vi "Registration Console.vi"(7 "Module Name":string="Module") -> ()   [LabVIEW 2017, in "DebugConsole.lvlib"]
uses:
  DebugConsole.lvlib
  _csmlite/_PassAllowedMessage - Mapping.vi
  _Polymophic/Build Unregister Message.vi
  _csmlite/_csmlite.lvlib
  Communicable State Machine.lvlib
  _ui/csm-ui-support.lvlib
panel:
  in  "Drop All":bool
  in  "Type":enum32{"Rules", "Mapping"}(radio)
  in  "Refresh API":bool
  out "RegistryList":string[][](table)
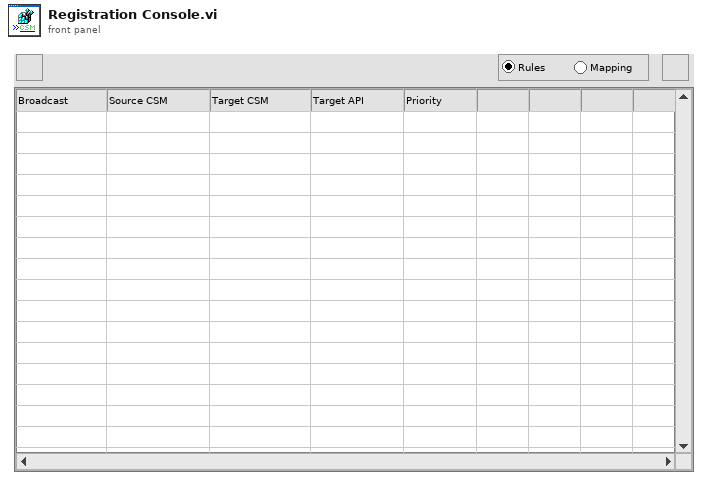
[diagram p1: front panel]
types:
  T1 = enum32{"Invalid", "Standard", "Closed", "Hidden", "Minimized", "Maximized"}
  T2 = enum32{"invalid app kind", "Development System", "Run Time System", "Student Edition", "Embedded LabVIEW", "Evaluation", "Custom"}
  T3 = typedef "LVPoint32TypeDef.ctl" = cluster{"Horizontal":i32, "Vertical":i32}
  T4 = typedef "LVRowAndColumnTypeDef.ctl" = cluster{"Row":i32, "Column":i32}
  T5 = cluster{"Core":cluster{"Current VI Reference":refnum<vi>, "Close Panel on Exit?":bool}, "Your Boolean data":bool, "Your string data":string}
  T6 = cluster{"Current VI Reference":refnum<vi>, "Close Panel on Exit?":bool}
  T7 = typedef "Communicable State Machine.lvlib/CSM - Broadcast Message Type.ctl" = enum16{"<Null>", "Status", "Interrupt"}
  T8 = cluster{"Status":string, "Source CSM":string, "Target CSM":string, "Target API":string, "Register Type":T7}[]
  T9 = cluster{string, "Name":string, "Target CSM":string, "Target State":string, "Register Type":T7}[]
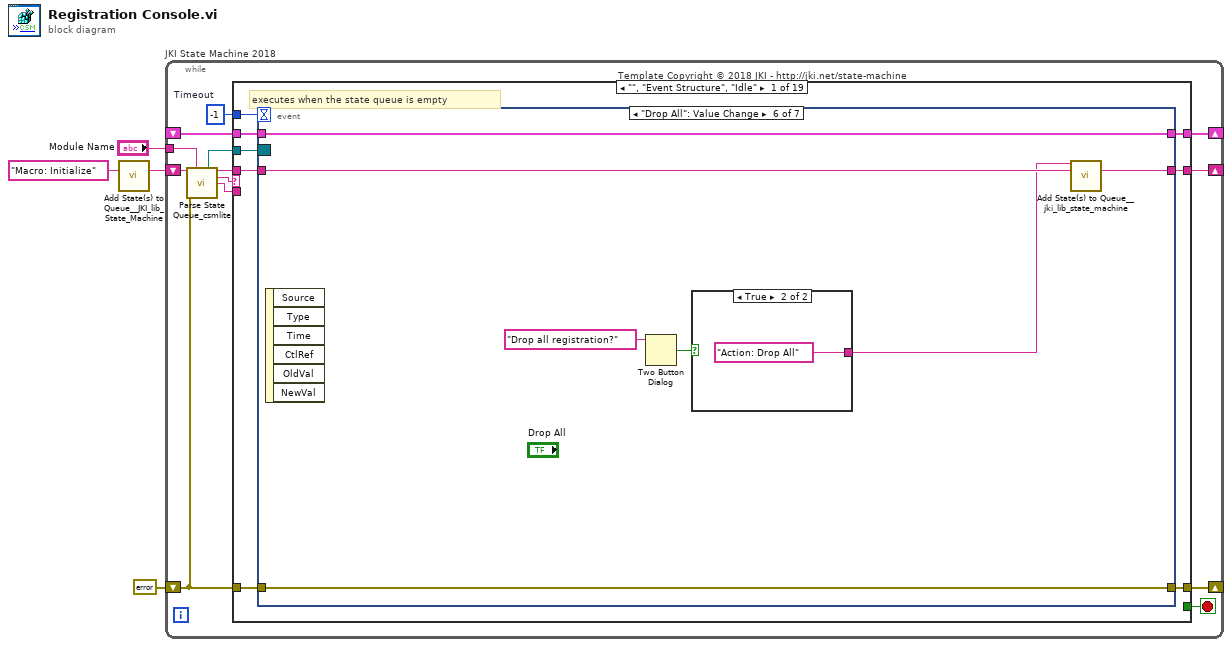
[diagram p0: block diagram]
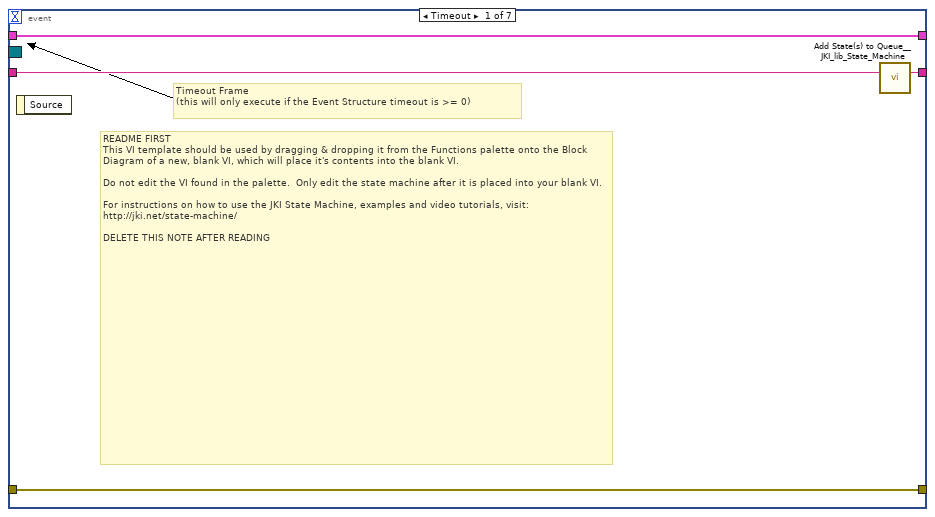
[diagram p2: hidden frame]
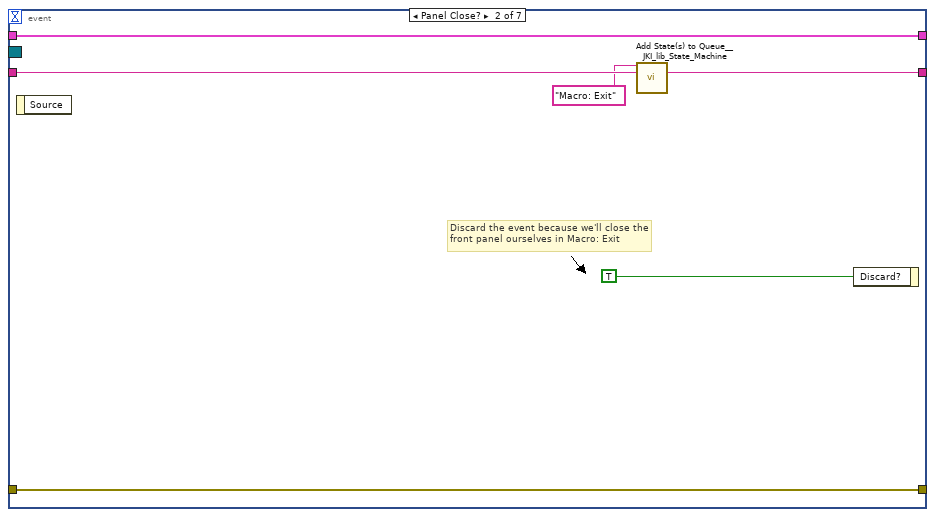
[diagram p3: hidden frame]
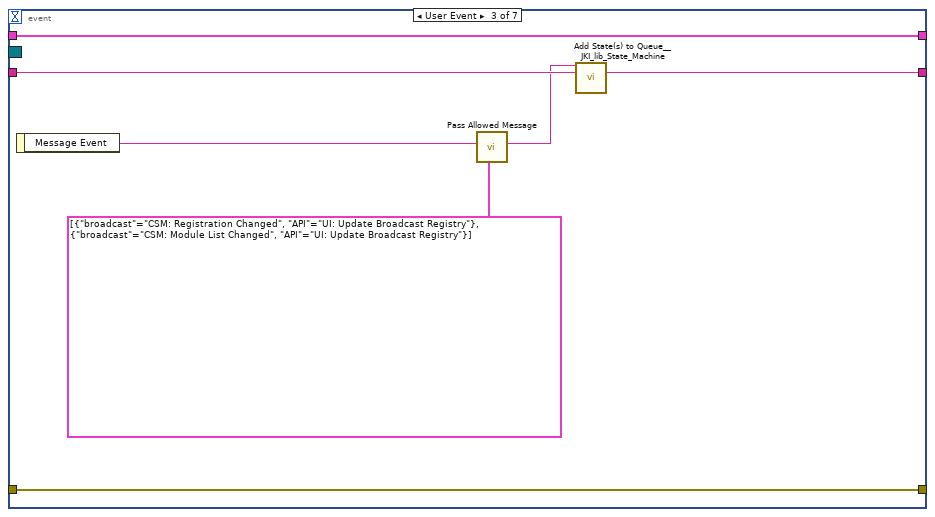
[diagram p4: hidden frame]
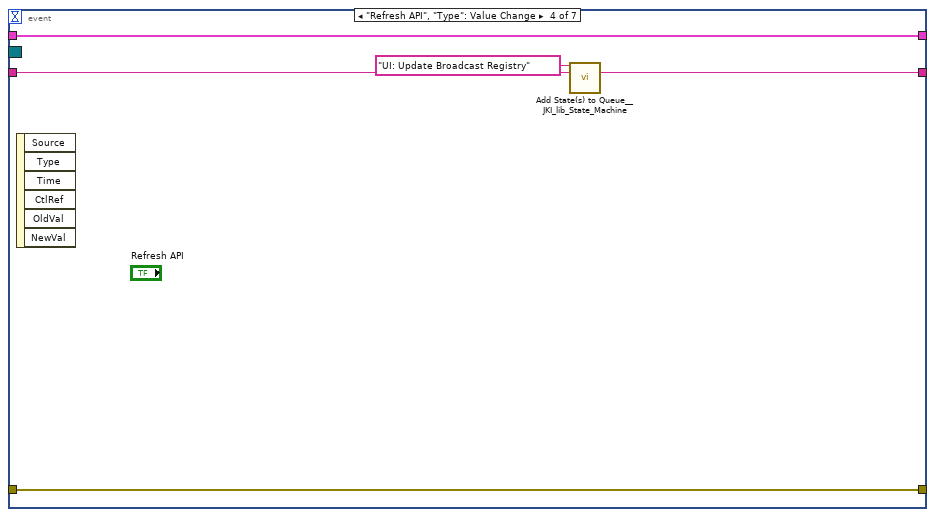
[diagram p5: hidden frame]
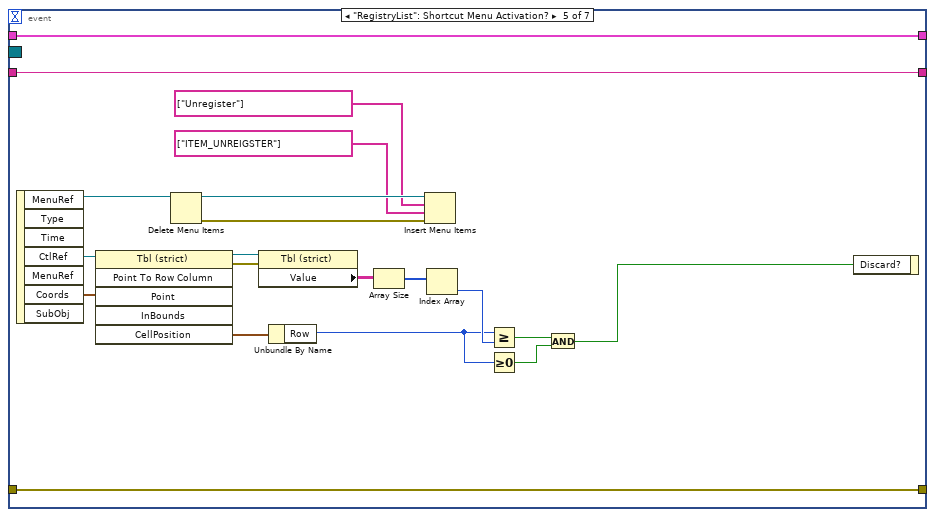
[diagram p6: hidden frame]
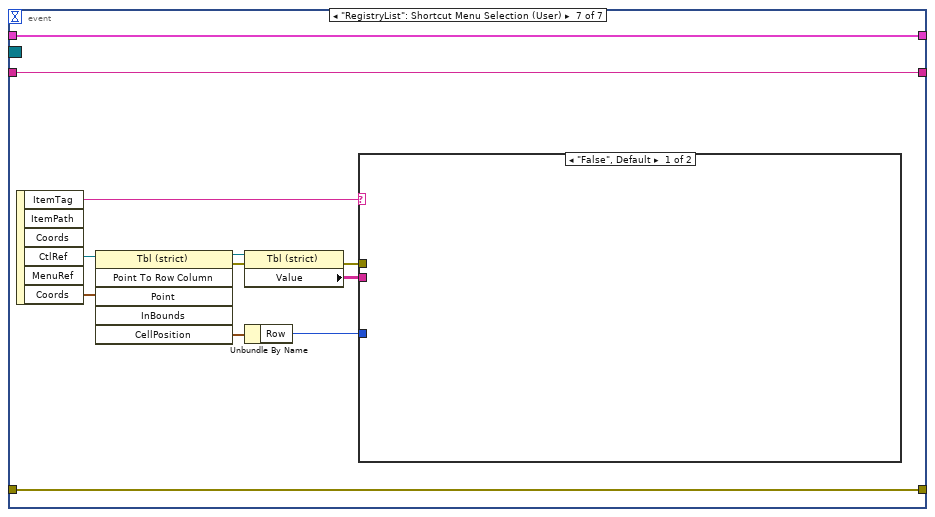
[diagram p8: hidden frame]
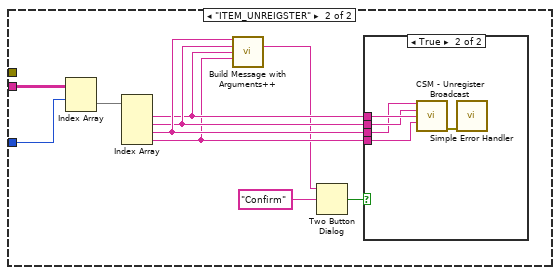
[diagram p9: hidden frame]
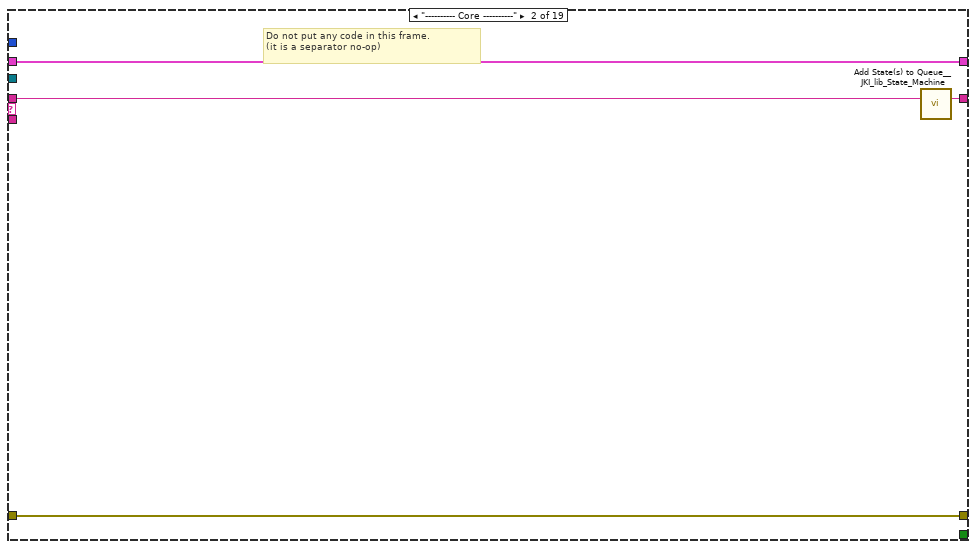
[diagram p11: hidden frame]
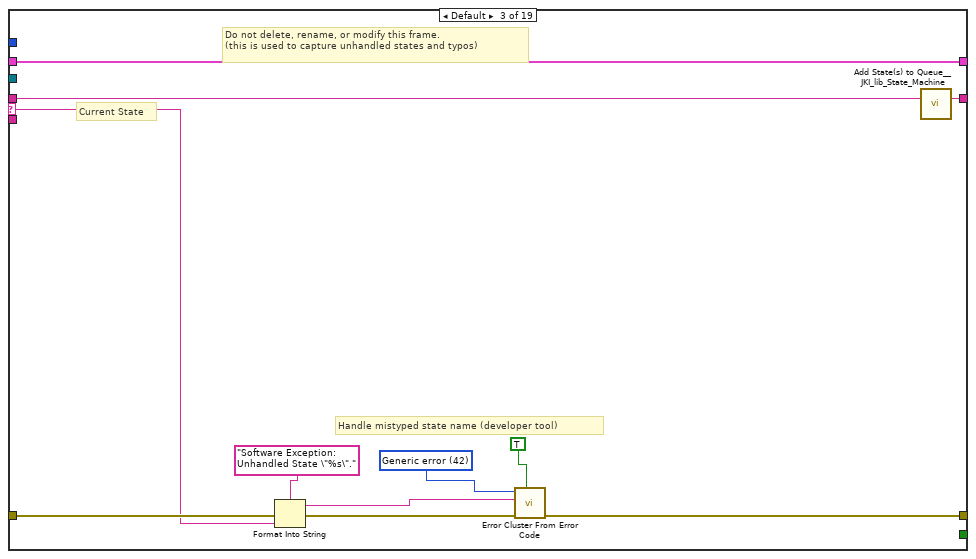
[diagram p12: hidden frame]
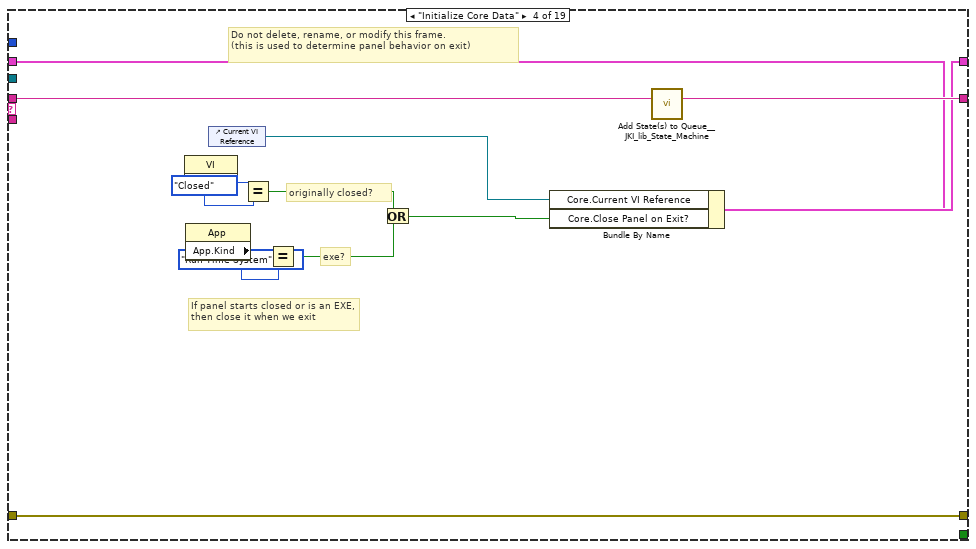
[diagram p13: hidden frame]
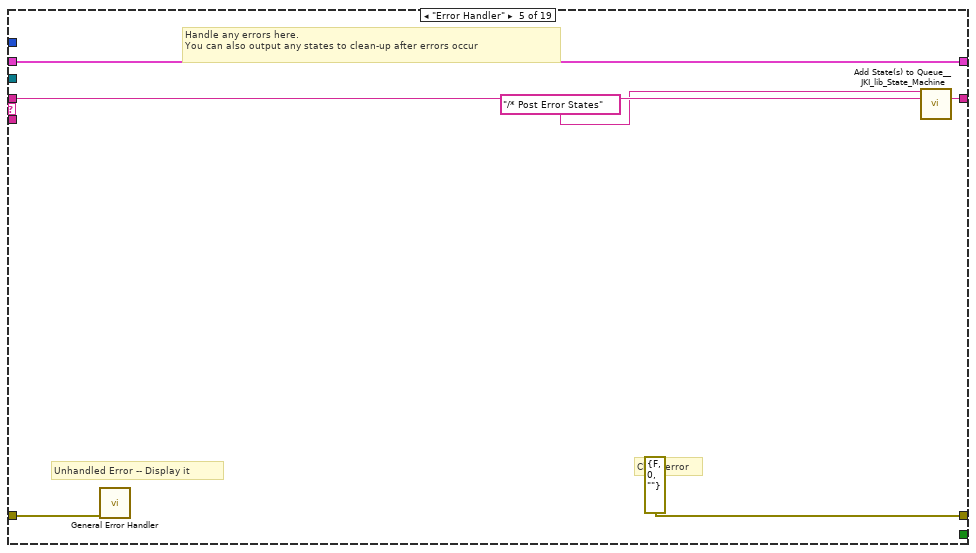
[diagram p14: hidden frame]
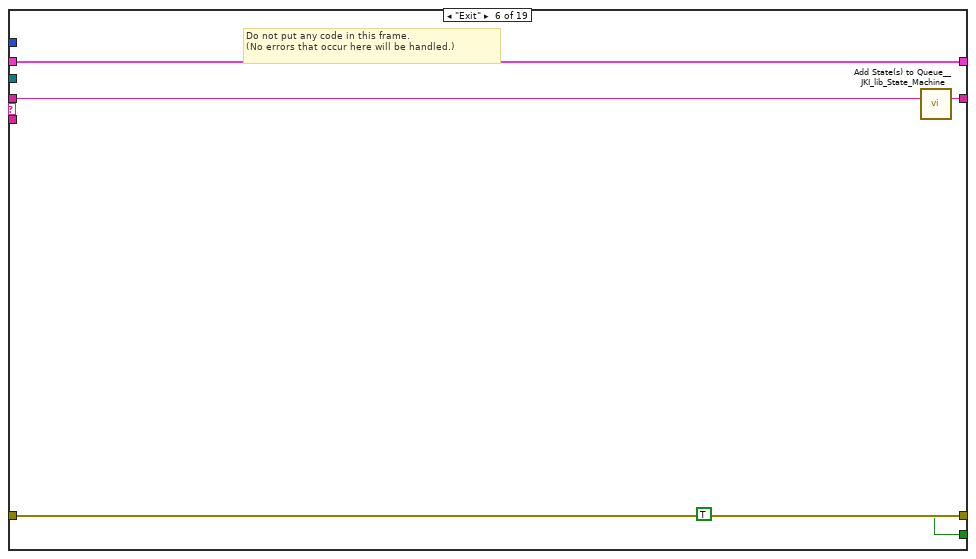
[diagram p15: hidden frame]
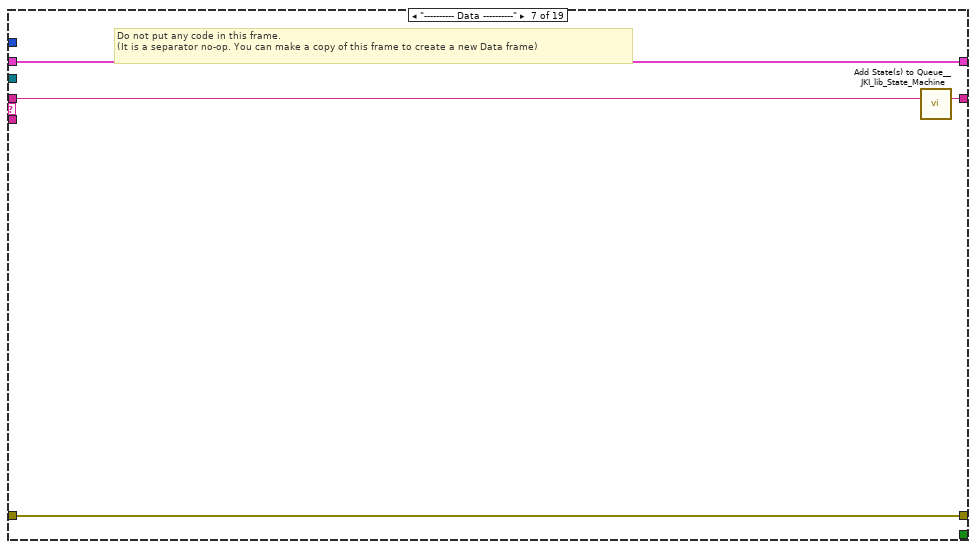
[diagram p16: hidden frame]
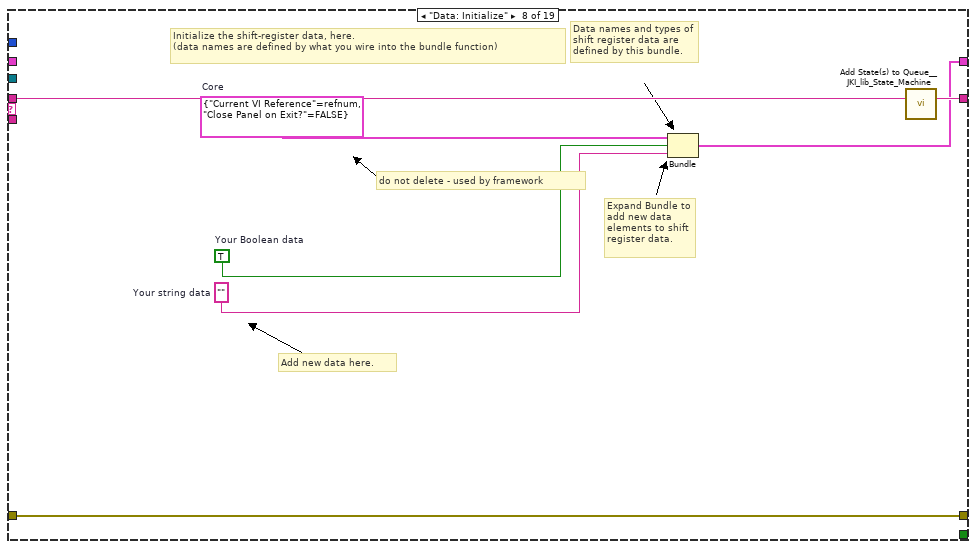
[diagram p17: hidden frame]
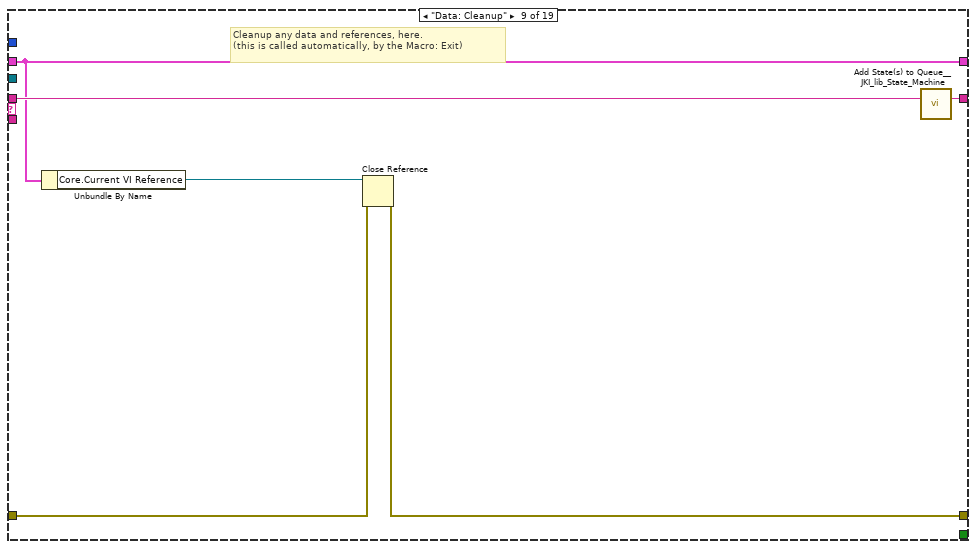
[diagram p18: hidden frame]
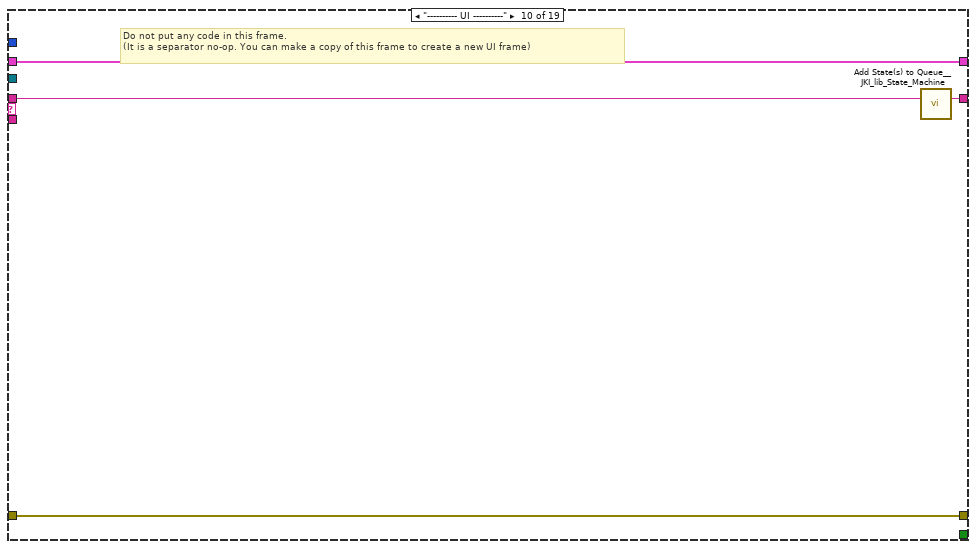
[diagram p19: hidden frame]
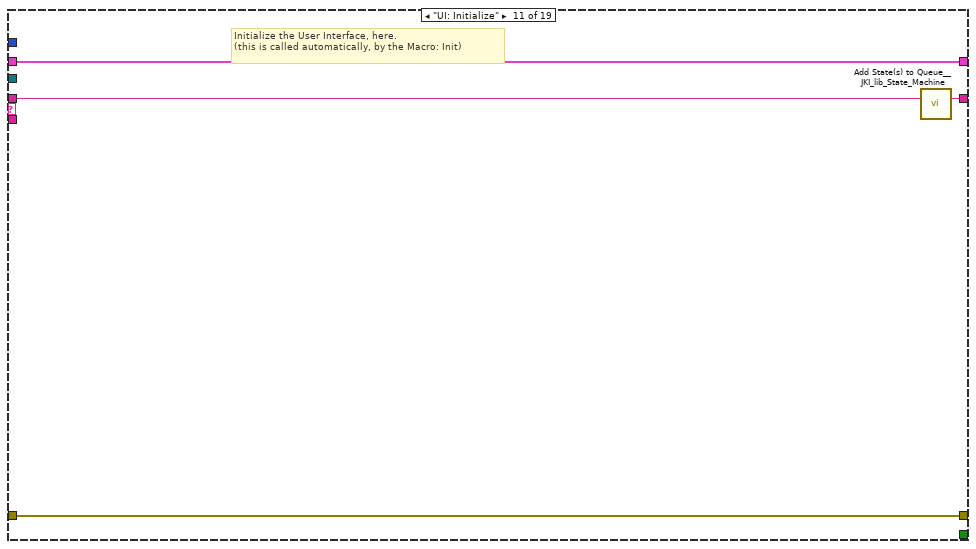
[diagram p20: hidden frame]
diagram:
  n1 = call <vilib>:"Add State(s) to Queue__JKI_lib_State_Machine.vi"("State(s) in (\"\")"="Macro: Initialize") -> ("States Out"=w3:string)  [unwired: 14 in]
  n2 = while "JKI State Machine 2018" {
    shift-right: [w10] -> _
    shift-left: _ -> [w9]
    shift-right: [w13] -> _
    shift-left: errorcluster {"status"=FALSE, "code"=0, "source"=""} ("error out") -> [w7]
    shift-right: [w12] -> _
    shift-left: w3 -> [w14]
    tunnel: "Module Name" -> [w6]
    stop <- w11 stop-if-true
    w8 = -1  # Timeout
    # "Template Copyright © 2018 JKI - http://jki.net/state-machine"
    n3 = call "Parse State Queue_csmlite.vi"("State Queue"=w14, "Current Module(\"\" to generate an ID)"=w6, "Error In (no error)"=w7) -> ("Event Registration Refnum"=w5:refnum<event-registration>, "Remaining States"=w16:string, "Current State"=w17:string, "Arguments"=w15:string)  [unwired: 9 in]
    n4 = case shown="\"\", \"Event Structure\", \"Idle\"" w17 {
      selector: w17 -> [_ _ w107 _ _ _ _ _ _ _ _ _ _ _ _ _ _ _ _]
      tunnel: w16 -> [w25 w106 w111 w130 w136 w141 w145 w152 w158 w162 w166 w172 w183 w259 w273 w278 w288 w292 w294]
      tunnel: w15 -> [_ _ _ _ _ _ _ _ _ _ _ w167 w177 _ _ _ _ _ _]
      tunnel: w9 -> [w23 w103 w109 w123 w133 w139 w142 _ w153 w159 w164 w170 w179 w256 w270 w275 w285 w289 w293]
      tunnel: [w22 w104 w113 w127 errorcluster {"status"=FALSE, "code"=0, "source"=""} ("error out") w138 w143 w149 w154 w160 w163 w168 w180 w257 w271 w276 w286 w290 w295] -> w13
      tunnel: w7 -> [w21 w104 w112 w127 w132 w138 w143 w149 w155 w160 w163 w169 w181 w257 w271 w276 w286 w290 w295]
      tunnel: [w24 w105 w110 w129 w135 w140 w144 w151 w157 w161 w165 w171 w182 w258 w272 w277 w287 w291 w294] -> w12
      tunnel: [_ _ _ _ _ TRUE _ _ _ _ _ _ _ _ _ _ _ _ _] -> w11
      tunnel: [w20 w103 w109 w128 w133 w139 w142 w150 w153 w159 w164 w170 w179 w256 w270 w275 w285 w289 w293] -> w10
      tunnel: w8 -> [w19 _ _ _ _ _ _ _ _ _ _ _ _ _ _ _ _ _ _]
      tunnel: w5 -> [w18 _ _ _ _ _ _ _ _ _ _ _ _ _ _ _ _ _ _]
      frame "", "Event Structure", "Idle" {
        # "executes when the state queue is empty"
        n5 = event shown="[5] \"Drop All\": Value Change" {
          selector: w18 -> [_ _ _ _ _ _ _]
          dyn-events: _ -> [_ _ _ _ _ _ _]
          timeout: w19 -> [_ _ _ _ _ _ _]
          tunnel: w25 -> [w29 w35 w40 w44 w67 w71 w87]
          tunnel: [w28 w34 w38 w45 w67 w72 w87] -> w24
          tunnel: w23 -> [w26 w32 w41 w46 w65 w73 w85]
          tunnel: [w27 w33 w42 w47 w66 w74 w86] -> w22
          tunnel: w21 -> [w27 w33 w42 w47 w66 w74 w86]
          tunnel: [w26 w32 w41 w46 w65 w73 w85] -> w20
          event Timeout {
            # "README FIRST\nThis VI template should be used by dragging & dropping it from the Functions palette onto the Block Diagram of a new, blank VI, which will place it's contents into the blank VI.\n\nDo not edit the VI found in the palette.  Only edit the state machine after it is placed into your blank VI.\n\nFor instructions on how to use the JKI State Machine, examples and video tutorials, visit:\nhttp://jki.net/state-machine/\n\nDELETE THIS NOTE AFTER READING"
            # "Timeout Frame\n(this will only execute if the Event Structure timeout is >= 0)"
            n6 = event-data() -> ()  [unwired: 1 in, 1 out]
            n7 = call <vilib>:"Add State(s) to Queue__JKI_lib_State_Machine.vi"("State(s) in (\"\")"=w29) -> ("States Out"=w28:string)  [unwired: 14 in]
          }
          event Panel Close? {
            # "Discard the event because we'll close the front panel ourselves in Macro: Exit"
            n8 = event-data() -> ()  [unwired: 1 in, 1 out]
            n9 = call <vilib>:"Add State(s) to Queue__JKI_lib_State_Machine.vi"("State(s) in Front (\"\")"="Macro: Exit", "State(s) in (\"\")"=w35) -> ("States Out"=w34:string)  [unwired: 13 in]
            n10 = event-data("Discard?"=TRUE) -> ()  [unwired: 1 in, 1 out]
          }
          event User Event {
            n11 = event-data() -> ("Message Event"=w39:string)  [unwired: 1 in]
            n12 = call-poly "Pass Allowed Message.vi"("Mapping"=cluster{"broadcast":string, "API":string}[] [{"broadcast"="CSM: Registration Changed", "API"="UI: Update Broadcast Registry"}, {"broadcast"="CSM: Module List Changed", "API"="UI: Update Broadcast Registry"}], "JKISM External Event"=w39) -> ("States"=w37:string)  [unwired: 7 in]
            n13 = call <vilib>:"Add State(s) to Queue__JKI_lib_State_Machine.vi"("State(s) in Front (\"\")"=w37, "State(s) in (\"\")"=w40) -> ("States Out"=w38:string)  [unwired: 13 in]
          }
          event "Refresh API", "Type": Value Change {
            n14 = event-data() -> ()  [unwired: 1 in, 6 out]
            n15 = call <vilib>:"Add State(s) to Queue__JKI_lib_State_Machine.vi"("State(s) in Front (\"\")"="UI: Update Broadcast Registry" ("State(s) in Front (\"\")"), "State(s) in (\"\")"=w44) -> ("States Out"=w45:string)  [unwired: 13 in]
          }
          event "RegistryList": Shortcut Menu Activation? {
            n16 = event-data() -> ("MenuRef"=w58:refnum<k9>, "CtlRef"=w64:refnum<vi>, "Coords"=w63:T3)  [unwired: 1 in, 4 out]
            n17 = invoke class="Tbl (strict)" method="Point To Row Column"(reference=w64, "Point"=w63) -> (reference out=w62:refnum<vi>, error out=w61:errorcluster, "CellPosition"=w60:T4)  [unwired: 4 in, 3 out]
            n18 = Delete Menu Items(9:w58) -> (0:w57:errorcluster, 3:w56:refnum<k9>)  [unwired: 3 in]
            n19 = property class="Tbl (strict)"(reference=w62, error in=w61) -> ("Value"=w59:string[][])  [unwired: 2 out]
            n20 = Unbundle By Name(w60) -> ("Row"=w49:i32)
            n21 = Array Size(array=w59) -> (size(s)=w53:i32[])
            n22 = Insert Menu Items(6:w57, 7:string[] ["ITEM_UNREIGSTER"] ("item names"), 8:string[] ["Unregister"] ("item names"), 9:w56) -> ()  [unwired: 2 in, 3 out]
            n23 = Index Array(array=w53) -> (element=w52:i32)  [unwired: 1 in]
            n24 = Greater Or Equal?(x=w49, y=w52) -> (x >= y?=w51:bool)
            n25 = Greater Or Equal To 0?(x=w49) -> (x >= 0?=w48:bool)
            n26 = And(x=w51, y=w48) -> (x .and. y?=w50:bool)
            n27 = event-data("Discard?"=w50) -> ()  [unwired: 1 in, 1 out]
          }
          event "Drop All": Value Change {
            n28 = event-data() -> ()  [unwired: 1 in, 6 out]
            n29 = Two Button Dialog(message="Drop all registration?") -> (T button?=w69:bool)  [unwired: 2 in]
            n30 = case shown="True" w69 {
              tunnel: [_ "Action: Drop All" ("State(s) in Front (\"\")")] -> w70
              frame False {
              }
              frame True {
              }
            }
            n31 = call <vilib>:"Add State(s) to Queue__jki_lib_state_machine.vi"("State(s) in Front (\"\")"=w70, "State(s) in (\"\")"=w71) -> ("States Out"=w72:string)  [unwired: 13 in]
          }
          event "RegistryList": Shortcut Menu Selection (User) {
            n32 = event-data() -> ("ItemTag"=w79:string, "CtlRef"=w84:refnum<vi>, "Coords"=w83:T3)  [unwired: 1 in, 3 out]
            n33 = invoke class="Tbl (strict)" method="Point To Row Column"(reference=w84, "Point"=w83) -> (reference out=w82:refnum<vi>, error out=w81:errorcluster, "CellPosition"=w80:T4)  [unwired: 4 in, 3 out]
            n34 = property class="Tbl (strict)"(reference=w82, error in=w81) -> (error out=w78:errorcluster, "Value"=w77:string[][])  [unwired: 1 out]
            n35 = Unbundle By Name(w80) -> ("Row"=w76:i32)
            n36 = case shown="\"False\", Default" w79 {
              tunnel: w78 -> [_ _]
              tunnel: w77 -> [_ w97]
              tunnel: w76 -> [_ w96]
              frame "False", Default {
              }
              frame "ITEM_UNREIGSTER" {
                n37 = Index Array(array=w97, index (row)=w96) -> (element=w95:string[])  [unwired: 1 in]
                n38 = Index Array(array=w95) -> (element #1=w91:string, element #2=w92:string, element #3=w93:string, element #4=w90:string)  [unwired: 4 in]
                n39 = call-poly "Build Message with Arguments++.vi"("Target CSM"=w93, "Source CSM (* as Default)"=w92, "Status"=w91, "API (* as Default)"=w90) -> ("CSM Message String"=w88:string)  [unwired: 11 in]
                n40 = Two Button Dialog(message=w88, 2:"Confirm" ("message")) -> (T button?=w94:bool)  [unwired: 1 in]
                n41 = case shown="True" w94 {
                  tunnel: w91 -> [_ w101]
                  tunnel: w92 -> [_ w100]
                  tunnel: w93 -> [_ w99]
                  tunnel: w90 -> [_ w98]
                  frame False {
                  }
                  frame True {
                    n42 = call "CSM - Unregister Broadcast.vi"("CSM Name(Empty for Broadcast Event)"=w99, "Source CSM Name (* as Default)"=w100, "Trigger"=w101, "API (\"*\" as Default)"=w98) -> ("error out"=w102:errorcluster)  [unwired: 10 in, 1 out]
                    n43 = call <vilib>:"Simple Error Handler.vi"("error in (no error)"=w102) -> ()  [unwired: 4 in, 5 out]
                  }
                }
              }
            }
          }
        }
      }
      frame "---------- Core ----------" {
        # "Do not put any code in this frame.\n(it is a separator no-op)"
        n44 = call <vilib>:"Add State(s) to Queue__JKI_lib_State_Machine.vi"("State(s) in (\"\")"=w106) -> ("States Out"=w105:string)  [unwired: 14 in]
      }
      frame Default {
        w116 = 42 items=["No error", "Argument error", "Memory is full", "Out of zone", "End of file", "File already open", "Generic file I/O error", "File not found", "File permission error", "Disk is full", "Duplicate path", "Too many files open", "System feature not enabled", "Resource file not found", "Cannot add resource", "Resource not found", "Image not found", "Image memory error", "Pen does not exist", "Config type invalid", "Config token not found", "Config parse error", "Config memory error", "Bad external code format", "Bad external code offset", "External code not present", "Null window", "Destroy window error", "Null menu", "Print aborted", "Bad print record", "Print driver error", "Windows error during printing", "Memory error during printing", "Print dialog error", "Generic print error", "Invalid device refnum", "Device not found", "Device parameter error", "Device unit error", "Cannot open device", "Device call aborted", "Generic error", "Cancelled by user", "Object ID too low", "Object ID too high", "Object not in heap", "Unknown heap", "Unknown object (invalid DefProc)", "Unknown object (DefProc not in table)", "Message out of range", "Invalid (null) method", "Unknown message", "Manager call not supported", "Bad address", "Network operation in progress", "Network operation timed out", "Connection is busy", "Network attribute not supported", "Network error", "Address in use", "System out of memory", "Connection aborted", "Connection refused", "Not connected", "Already connected", "Connection closed", "Initialization error (interapplication manager)", "Bad occurrence", "Wait on unbound occurrence handler", "Occurrence queue overflow", "Datalog type conflict", "Unused", "Unrecognized type (interapplication manager)", "Memory corrupt", "Failed to make temporary DLL", "Old CIN version", "Drag socket not found", "Failed to load drop-object", "Failed to register OLE object", "Failed to release OLE object", "Format specifier type mismatch", "Unknown format specifier", "Too few format specifiers", "Too many format specifiers", "Scan failed", "Newer CIN version", "Error converting to variant", "Runtime menu error", "Password tampered", "Variant attribute not found", "Incompatible variant data type", "Event data is not available", "Event Store is not present", "Occurrence is not found", "Event Queue is not created", "Event info is not available", "Refnum passed is NULL", "Error retrieving Class GUID", "Error retrieving CoClass GUID", "Error retrieving TypeLib GUID.", "Bad built application magic bytes.", "Specific driver is different from the specific driver associated with the Logical Name.", "There is no session opened to the class driver.", "Max Error", "MAX - Error with config objects", "MAX - Error loading configuration", "MAX - Group not supported"]
        # "Current State"
        # "Do not delete, rename, or modify this frame.\n(this is used to capture unhandled states and typos)"
        # "Handle mistyped state name (developer tool)"
        n45 = Format Into String(format string="Software Exception: Unhandled State \"%s\"." ("message"), error in=w112, w107) -> (resulting string=w115:string, error out=w114:errorcluster)  [unwired: 1 in]
        n46 = call <vilib>:"Error Cluster From Error Code.vi"("show call chain? (False)"=TRUE, "error in (no error)"=w114, "error message (\"\")"=w115, "error code (0)"=w116) -> ("error out"=w113:errorcluster)  [unwired: 5 in]
        n47 = call <vilib>:"Add State(s) to Queue__JKI_lib_State_Machine.vi"("State(s) in (\"\")"=w111) -> ("States Out"=w110:string)  [unwired: 14 in]
      }
      frame "Initialize Core Data" {
        # "Do not delete, rename, or modify this frame.\n(this is used to determine panel behavior on exit)"
        # "originally closed?"
        # "exe?"
        # "If panel starts closed or is an EXE, then close it when we exit"
        n48 = property class="VI"() -> ("FP.State"=w120:T1)  [unwired: 2 in, 2 out]
        n49 = property class="App"() -> ("App.Kind"=w126:T2)  [unwired: 2 in, 2 out]
        n50 = control-ref of="Current VI Reference"() -> (w121:refnum<vi>)
        n51 = Equal?(x=w120, y=T1."Closed" ("Front Panel Window:State")) -> (x = y?=w118:bool)
        n52 = Equal?(x=w126, y=T2."Run Time System" ("Application:Kind")) -> (x = y?=w124:bool)
        n53 = Or(x=w118, y=w124) -> (x .or. y?=w122:bool)
        n54 = Bundle By Name(cluster=w123, "Core.Current VI Reference"=w121, "Core.Close Panel on Exit?"=w122) -> (w128:T5)
        n55 = call <vilib>:"Add State(s) to Queue__JKI_lib_State_Machine.vi"("State(s) in (\"\")"=w130) -> ("States Out"=w129:string)  [unwired: 14 in]
      }
      frame "Error Handler" {
        # "Unhandled Error -- Display it"
        # "Handle any errors here.\nYou can also output any states to clean-up after errors occur"
        # "Clear error"
        n56 = call <vilib>:"General Error Handler.vi"("error in (no error)"=w132) -> ()  [unwired: 10 in, 5 out]
        n57 = call <vilib>:"Add State(s) to Queue__JKI_lib_State_Machine.vi"("State(s) in Front (\"\")"="/* Post Error States", "State(s) in (\"\")"=w136) -> ("States Out"=w135:string)  [unwired: 13 in]
      }
      frame "Exit" {
        # "Do not put any code in this frame.\n(No errors that occur here will be handled.)"
        n58 = call <vilib>:"Add State(s) to Queue__JKI_lib_State_Machine.vi"("State(s) in (\"\")"=w141) -> ("States Out"=w140:string)  [unwired: 14 in]
      }
      frame "---------- Data ----------" {
        # "Do not put any code in this frame.\n(It is a separator no-op. You can make a copy of this frame to create a new Data frame)"
        n59 = call <vilib>:"Add State(s) to Queue__JKI_lib_State_Machine.vi"("State(s) in (\"\")"=w145) -> ("States Out"=w144:string)  [unwired: 14 in]
      }
      frame "Data: Initialize" {
        w146 = T6 {"Current VI Reference"=refnum, "Close Panel on Exit?"=FALSE}  # Core
        w148 = TRUE  # Your Boolean data
        w147 = ""  # Your string data
        # "do not delete - used by framework"
        # "Expand Bundle to add new data elements to shift register data."
        # "Add new data here."
        # "Data names and types of shift register data are defined by this bundle."
        # "Initialize the shift-register data, here.\n(data names are defined by what you wire into the bundle function)"
        n60 = Bundle("Core"=w146, "Your Boolean data"=w148, "Your string data"=w147) -> (w150:T5)  [unwired: 1 in]
        n61 = call <vilib>:"Add State(s) to Queue__JKI_lib_State_Machine.vi"("State(s) in (\"\")"=w152) -> ("States Out"=w151:string)  [unwired: 14 in]
      }
      frame "Data: Cleanup" {
        # "Cleanup any data and references, here.\n(this is called automatically, by the Macro: Exit)"
        n62 = Unbundle By Name(w153) -> ("Core.Current VI Reference"=w156:refnum<vi>)
        n63 = Close Reference(reference=w156, error in (no error)=w155) -> (error out=w154:errorcluster)
        n64 = call <vilib>:"Add State(s) to Queue__JKI_lib_State_Machine.vi"("State(s) in (\"\")"=w158) -> ("States Out"=w157:string)  [unwired: 14 in]
      }
      frame "---------- UI ----------" {
        # "Do not put any code in this frame.\n(It is a separator no-op. You can make a copy of this frame to create a new UI frame)"
        n65 = call <vilib>:"Add State(s) to Queue__JKI_lib_State_Machine.vi"("State(s) in (\"\")"=w162) -> ("States Out"=w161:string)  [unwired: 14 in]
      }
      frame "UI: Initialize" {
        # "Initialize the User Interface, here.\n(this is called automatically, by the Macro: Init)"
        n66 = call <vilib>:"Add State(s) to Queue__JKI_lib_State_Machine.vi"("State(s) in (\"\")"=w166) -> ("States Out"=w165:string)  [unwired: 14 in]
      }
      frame "UI: Cursor Set" {
        # "Argument"
        # "Set and Unset Cursor Busy.\n(Usage: \"UI: Cursor Set >> Busy|Idle\")"
        n67 = case shown="\"Idle\", Default" w167 {
          tunnel: w169 -> [w174 w176]
          tunnel: [w173 w175] -> w168
          frame "Idle", Default {
            n68 = call <vilib>:"Unset Busy.vi"("error in (no error)"=w174) -> ("error out"=w173:errorcluster)  [unwired: 10 in]
          }
          frame "Busy" {
            n69 = call <vilib>:"Set Busy.vi"("error in (no error)"=w176) -> ("error out"=w175:errorcluster)  [unwired: 9 in, 1 out]
          }
        }
        n70 = call <vilib>:"Add State(s) to Queue__JKI_lib_State_Machine.vi"("State(s) in (\"\")"=w172) -> ("States Out"=w171:string)  [unwired: 14 in]
      }
      frame "UI: Front Panel State" {
        # "Argument"
        # "Set Front Panel Open or Closed\n(Usage: \"UI: Front Panel State >> Open|Close\")"
        n71 = Unbundle By Name(w179) -> ("Core.Current VI Reference"=w178:refnum<vi>)
        n72 = case shown="\"Minimize\", \"Minimized\"" w177 {
          tunnel: w181 -> [w189 w204 w215 w228 w241]
          tunnel: [w191 w205 w217 w230 w243] -> w180
          tunnel: w178 -> [w190 w202 w216 w229 w242]
          frame "Open", "Standard", Default {
            w184 = T1."Standard" ("State")
            n73 = property class="VI"(reference=w190, error in=w189) -> (reference out=w187:refnum<vi>, error out=w188:errorcluster, "FP.State"=w186:T1)
            n74 = Not Equal?(x=w186, y=w184) -> (x != y?=w185:bool)
            n75 = case shown="True" w185 {
              tunnel: [w195 w197] -> w191
              tunnel: w188 -> [w194 w197]
              tunnel: w187 -> [w193 _]
              tunnel: w184 -> [w192 _]
              frame True {
                n76 = invoke class="VI" method="FP.Open"(reference=w193, error in=w194, "Activate"=TRUE, "State"=w192) -> (error out=w195:errorcluster)  [unwired: 1 in, 4 out]
              }
              frame False {
              }
            }
          }
          frame "Close", "Closed" {
            n77 = property class="VI"(reference=w202, error in=w204) -> (reference out=w201:refnum<vi>, error out=w203:errorcluster, "FP.State"=w199:T1)
            n78 = Not Equal?(x=w199, y=T1."Closed" ("Front Panel Window:State")) -> (x != y?=w198:bool)
            n79 = case shown="True" w198 {
              tunnel: [w206 w209] -> w205
              tunnel: w203 -> [w206 w208]
              tunnel: w201 -> [_ w207]
              frame False {
              }
              frame True {
                n80 = invoke class="VI" method="FP.Close"(reference=w207, error in=w208) -> (error out=w209:errorcluster)  [unwired: 1 in, 2 out]
              }
            }
          }
          frame "Hidden", "Hide" {
            w210 = T1."Hidden" ("State")
            n81 = property class="VI"(reference=w216, error in=w215) -> (reference out=w213:refnum<vi>, error out=w214:errorcluster, "FP.State"=w212:T1)
            n82 = Not Equal?(x=w212, y=w210) -> (x != y?=w211:bool)
            n83 = case shown="True" w211 {
              tunnel: [w221 w222] -> w217
              tunnel: w214 -> [w220 w222]
              tunnel: w213 -> [w219 _]
              tunnel: w210 -> [w218 _]
              frame True {
                n84 = invoke class="VI" method="FP.Open"(reference=w219, error in=w220, "State"=w218) -> (error out=w221:errorcluster)  [unwired: 2 in, 4 out]
              }
              frame False {
              }
            }
          }
          frame "Minimize", "Minimized" {
            w223 = T1."Minimized" ("State")
            n85 = property class="VI"(reference=w229, error in=w228) -> (reference out=w226:refnum<vi>, error out=w227:errorcluster, "FP.State"=w225:T1)
            n86 = Not Equal?(x=w225, y=w223) -> (x != y?=w224:bool)
            n87 = case shown="True" w224 {
              tunnel: [w234 w235] -> w230
              tunnel: w227 -> [w233 w235]
              tunnel: w226 -> [w232 _]
              tunnel: w223 -> [w231 _]
              frame True {
                n88 = invoke class="VI" method="FP.Open"(reference=w232, error in=w233, "State"=w231) -> (error out=w234:errorcluster)  [unwired: 2 in, 4 out]
              }
              frame False {
              }
            }
          }
          frame "Maximize", "Maximized" {
            w236 = T1."Maximized" ("State")
            n89 = property class="VI"(reference=w242, error in=w241) -> (reference out=w239:refnum<vi>, error out=w240:errorcluster, "FP.State"=w238:T1)
            n90 = Not Equal?(x=w238, y=w236) -> (x != y?=w237:bool)
            n91 = case shown="True" w237 {
              tunnel: [w247 w248] -> w243
              tunnel: w240 -> [w246 w248]
              tunnel: w239 -> [w245 _]
              tunnel: w236 -> [w244 _]
              frame True {
                n92 = invoke class="VI" method="FP.Open"(reference=w245, error in=w246, "State"=w244) -> (error out=w247:errorcluster)  [unwired: 2 in, 4 out]
              }
              frame False {
              }
            }
          }
        }
        n93 = call <vilib>:"Add State(s) to Queue__JKI_lib_State_Machine.vi"("State(s) in (\"\")"=w183) -> ("States Out"=w182:string)  [unwired: 14 in]
      }
      frame "UI: Update Broadcast Registry" {
        n94 = case shown="\"Rules\", Default" "Type" {
          tunnel: [w260 w261] -> w255
          frame "Rules", Default {
            n95 = call "CSM - List Rules in Broadcast Registry.vi"() -> ("Rule Entries with Register Type"=w260:T8)  [unwired: 9 in, 2 out]
          }
          frame "Mapping" {
            n96 = call "CSM - List Mapping Relationships in Broadcast Registry.vi"() -> ("Mapping Relationships"=w261:T9)  [unwired: 10 in, 1 out]
          }
        }
        n97 = for {
          tunnel: w255 -> [w269] mode=indexing
          tunnel: [w262] -> w254 mode=indexing
          n98 = Unbundle(w269) -> ("Status"=w268:string, "Name"=w267:string, "Target CSM"=w266:string, "Target State"=w265:string, "Register Type"=w264:T7)
          n99 = Format Into String(w264) -> (resulting string=w263:string)  [unwired: 3 in, 1 out]
          n100 = Build Array(w268, w267, w266, w265, w263) -> (w262:string[])
        }
        "RegistryList" <- w254
        n101 = control-ref of="RegistryList"() -> (w253:refnum<vi>)
        n102 = property class="Tbl (strict)"(reference=w253) -> (reference out=w251:refnum<vi>, "Column Headers[]"=w249:string[])  [unwired: 1 in, 1 out]
        n103 = Build Array (concatenate)(w254, w249) -> (w250:string[][])
        n104 = call "Auto Resize All MultiListbox Columns (Uniform Text).vi"("Array"=w250, "Control In"=w251) -> ()  [unwired: 9 in, 1 out]
        n105 = call <vilib>:"Add State(s) to Queue__JKI_lib_State_Machine.vi"("State(s) in (\"\")"=w259) -> ("States Out"=w258:string)  [unwired: 14 in]
      }
      frame "---------- Macro ----------" {
        # "Do not put any code in this frame.\n(It is a separator no-op. You can make a copy of this frame to create a new Macro frame)"
        n106 = call <vilib>:"Add State(s) to Queue__JKI_lib_State_Machine.vi"("State(s) in (\"\")"=w273) -> ("States Out"=w272:string)  [unwired: 14 in]
      }
      frame "Macro: Initialize" {
        # "Initialization Macro\n(This is called once, when the VI starts)"
        n107 = call <vilib>:"Add State(s) to Queue__JKI_lib_State_Machine.vi"("State(s) in Front (\"\")"="Data: Initialize\nInitialize Core Data\nUI: Initialize\nUI: Update Broadcast Registry", "State(s) in (\"\")"=w278) -> ("States Out"=w277:string)  [unwired: 13 in]
      }
      frame "Macro: Exit" {
        # "Exit Macro\n(This is called once, when the VI exits)"
        n108 = Unbundle By Name(w285) -> ("Core.Close Panel on Exit?"=w284:bool)
        n109 = Select(t="UI: Front Panel State >> Close", s=w284, f="") -> (s? t:f=w281:string)
        n110 = call <vilib>:"Add State(s) to Queue__JKI_lib_State_Machine.vi"("State(s) in (\"\")"=w281, "State(s) at Back (\"\")"="Data: Cleanup\nExit") -> ("States Out"=w279:string)  [unwired: 13 in]
        n111 = call <vilib>:"Add State(s) to Queue__JKI_lib_State_Machine.vi"("State(s) in Front (\"\")"=w279, "State(s) in (\"\")"=w288) -> ("States Out"=w287:string)  [unwired: 13 in]
      }
      frame "---------- Action ----------" {
        # "Template Separator\n(You can make a copy of, or modify, this frame)"
        n112 = call <vilib>:"Add State(s) to Queue__JKI_lib_State_Machine.vi"("State(s) in (\"\")"=w292) -> ("States Out"=w291:string)  [unwired: 14 in]
      }
      frame "Action: Drop All" {
        n113 = call "CSM - Drop Broadcast Registry.vi"() -> ()  [unwired: 15 in, 1 out]
      }
    }
  }
